vi "UDP Ports.vi"() -> (1 "net address":u32, 2 "TX Port":u16, 3 "RX Port":u16=14550)   [LabVIEW 2014]
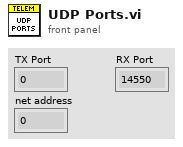
[diagram p1: front panel]
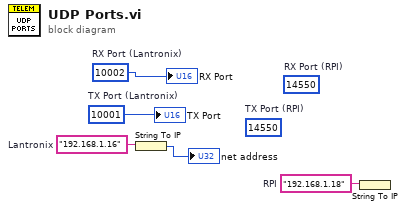
[diagram p0: block diagram]
diagram:
  w4 = "192.168.1.18"  # RPI
  w2 = u16 10001  # TX Port (Lantronix)
  w5 = "192.168.1.16"  # Lantronix
  w1 = u16 10002  # RX Port (Lantronix)
  (unwired) u16 14550  # TX Port (RPI)
  (unwired) u16 14550  # RX Port (RPI)
  n1 = String To IP(1:w5) -> (0:→"net address":u32)
  n2 = String To IP(1:w4) -> ()  [unwired: 1 out]
  "RX Port" <- w1
  "TX Port" <- w2
